vi "ADAM-4117_Log_ModbusRTU.NET.vi"() -> ()   [LabVIEW 2014]
uses:
  ModbusRTU/bin/Debug/Advantech.Adam.dll
  <vilib>/Platform/TimedLoop/XDataNode/timing_clust.ctl
  <vilib>/Platform/TimedLoop/XDataNode/nitl_modes.ctl
  <vilib>/Platform/TimedLoop/XDataNode/wakeup.ctl
  <vilib>/Platform/TimedLoop/XDataNode/XDataNode.xnode
  <vilib>/Platform/TimedLoop/XDataNode/XDNodeRunTimeDep.lvlib
panel:
  out "Waveform Chart":dbl(graph)
  out "ReadHoldingRegs":bool
  out "SetComPortTimeout":bool
  out "SetComPortState":bool
  out "OpenComPort":bool
  out "CloseComPort":bool
  in  "stop":bool
  in  "Address":i32=3
  in  "COM Port":i32=3
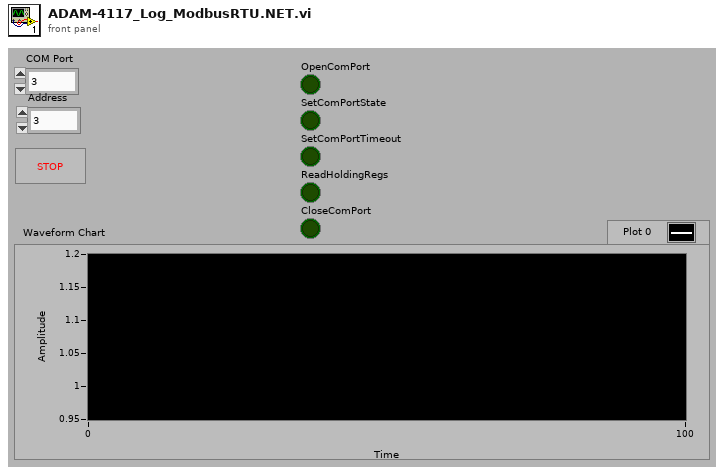
[diagram p1: front panel]
types:
  T1 = enum16{"open", "replace", "create", "open or create", "replace or create", "replace or create with confirmation"}
  T2 = typedef "XDNodeRunTimeDep.lvlib/timing_clust.ctl" = cluster{"Expected End [f-1]":u64, "Actual End [f-1]":u64, "Finished Late? [f-1]":bool, "Expected End [i-1]":u64, "Actual End [i-1]":u64, "Finished Late? [i-1]":bool, "Expected Start [i]":u64, "Actual Start [i]":u64, "Expected Start [f]":u64, "Actual Start [f]":u64, "Source Name":string, "Structure Name":string, "Period":i64, "Deadline":i64, "Offset":i64, "Start":i64, "Priority":i32, "Timeout":i32, "Mode":T3, "Wakeup Reason":T4, "Error":errorcluster, "Source Type":string, "Secondary Source Type":string, "Global End Time":u64, "Global Start Time":u64, "Frame Duration":u64, "Iteration Duration":u64, "Assigned CPU":i32, "I/O Scan Engine Mode":u32}
  T3 = typedef "XDNodeRunTimeDep.lvlib/nitl_modes.ctl" = enum32{"No Change", "Process missed periods, maintain original phase", "Discard missed periods, maintain original phase", "Process missed periods, ignore original phase", "Discard missed periods, ignore original phase"}
  T4 = typedef "XDNodeRunTimeDep.lvlib/wakeup.ctl" = enum32{"Normal", "Aborted", "Asynchronous wakeup", "Timing source error", "Timed loop error", "Timeout"}
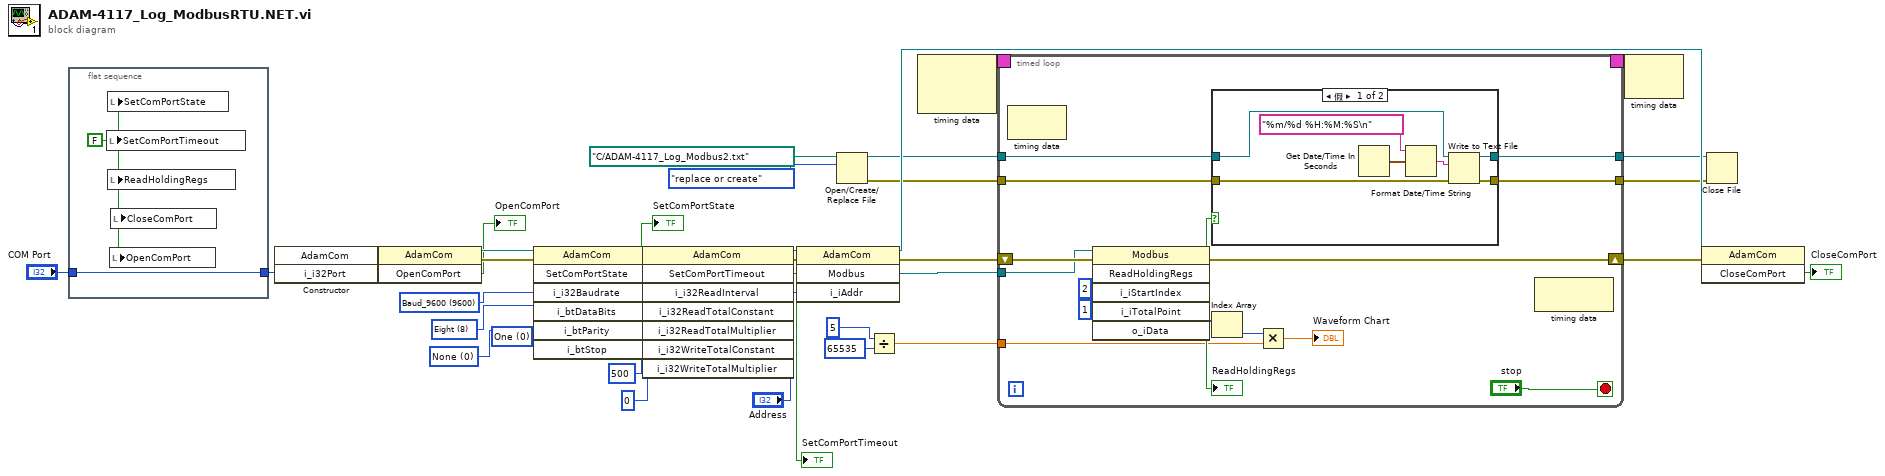
[diagram p0: block diagram]
diagram:
  w25 = 0 ("i_i32ReadTotalMultiplier")
  w26 = 500 ("i_i32ReadInterval")
  w29 = u8 0 items=["One", "OneAndHalf", "Two"] ("i_btStop")
  w30 = u8 0 items=["None", "Odd", "Even", "Mark", "Space"] ("i_btParity")
  w31 = u8 8 items=["Five"=5, "Six"=6, "Seven"=7, "Eight"=8] ("i_btDataBits")
  w32 = 9600 items=["Baud_110"=110, "Baud_300"=300, "Baud_600"=600, "Baud_1200"=1200, "Baud_2400"=2400, "Baud_4800"=4800, "Baud_9600"=9600, "Baud_14400"=14400, "Baud_19200"=19200, "Baud_38400"=38400, "Baud_56000"=56000, "Baud_57600"=57600, "Baud_115200"=115200, "Baud_128000"=128000, "Baud_256000"=256000] ("i_i32Baudrate")
  n1 = flat-sequence {
    tunnel: "COM Port" -> [w38]
    tunnel: [w38] -> w10
    frame #0 {
      w37 = FALSE
      n2 = local write "SetComPortTimeout"(w37) -> ()
      n3 = local write "SetComPortState"(w37) -> ()
      n4 = local write "ReadHoldingRegs"(w37) -> ()
      n5 = local write "OpenComPort"(w37) -> ()
      n6 = local write "CloseComPort"(w37) -> ()
    }
  }
  n7 = constructor class="AdamCom"("i_i32Port"=w10) -> (reference out=w36:refnum<k24>, error out=w35:errorcluster)  [unwired: 3 in, 2 out]
  n8 = invoke class="AdamCom" method="OpenComPort"(reference=w36, error in=w35) -> (reference out=w33:refnum<k24>, error out=w34:errorcluster, "OpenComPort"=→"OpenComPort":bool)  [unwired: 1 in]
  n9 = invoke class="AdamCom" method="SetComPortState"(reference=w33, error in=w34, "i_i32Baudrate"=w32, "i_btDataBits"=w31, "i_btParity"=w30, "i_btStop"=w29) -> (reference out=w27:refnum<k24>, error out=w28:errorcluster, "SetComPortState"=→"SetComPortState":bool)  [unwired: 1 in, 4 out]
  n10 = invoke class="AdamCom" method="SetComPortTimeout"(reference=w27, error in=w28, "i_i32ReadInterval"=w26, "i_i32ReadTotalConstant"=w26, "i_i32ReadTotalMultiplier"=w25, "i_i32WriteTotalConstant"=w26, "i_i32WriteTotalMultiplier"=w25) -> (reference out=w24:refnum<k24>, error out=w23:errorcluster, "SetComPortTimeout"=→"SetComPortTimeout":bool)  [unwired: 1 in, 5 out]
  n11 = invoke class="AdamCom" method="Modbus"(reference=w24, error in=w23, "i_iAddr"="Address") -> (reference out=w15:refnum<k24>, error out=w17:errorcluster, "Modbus"=w21:refnum<k24>)  [unwired: 1 in, 1 out]
  n12 = Open/Create/Replace File(file path (use dialog)=path "C:/ADAM-4117_Log_Modbus2.txt", operation (0:open)=T1."replace or create") -> (refnum out=w5:refnum<file>, error out=w7:errorcluster)  [unwired: 1 in, 4 out]
  n13 = Divide(x=5, y=65535) -> (x/y=w1:dbl)
  n14 = node-c288() -> (w20:T2)  [unwired: 2 out]
  n15 = timed-loop {
    timing: w20 -> [_]
    timing-out: [_] -> w19
    tunnel: w21 -> [w50]
    shift-right: [w51] -> w16
    shift-left: w17 -> [w52]
    tunnel: w7 -> [w46]
    tunnel: [w45] -> w6
    tunnel: w5 -> [w44]
    tunnel: [w43] -> w4
    tunnel: w1 -> [w40]
    stop <- "stop" stop-if-true
    n16 = node-c288() -> ()  [unwired: 2 out]
    n17 = invoke class="Modbus" method="ReadHoldingRegs"(reference=w50, error in=w52, "i_iStartIndex"=2, "i_iTotalPoint"=1) -> (error out=w51:errorcluster, "ReadHoldingRegs"=w42:bool, "o_iData"=w47:i32[])  [unwired: 2 in, 3 out]
    "ReadHoldingRegs" <- w42
    n18 = case shown="假" w42 {
      tunnel: w46 -> [w60 w62]
      tunnel: [w59 w62] -> w45
      tunnel: w44 -> [w58 w61]
      tunnel: [w57 w61] -> w43
      frame False {
        n19 = Get Date/Time In Seconds() -> (seconds since 1Jan1904=w54:timestamp)
        n20 = Format Date/Time String(time format string (%c)="%m/%d %H:%M:%S\n", seconds (now)=w54) -> (date/time string=w55:string)  [unwired: 1 out]
        n21 = Write to Text File(file (use dialog)=w58, text=w55, error in=w60) -> (refnum out=w57:refnum<file>, error out=w59:errorcluster)  [unwired: 2 out]
      }
      frame True {
      }
    }
    n22 = Index Array(array=w47) -> (element=w41:i32)  [unwired: 1 in]
    n23 = Multiply(x=w41, y=w40) -> (x*y=→"Waveform Chart":dbl)
    n24 = node-c288() -> ()  [unwired: 2 out]
  }
  n25 = node-c288(w19) -> ()  [unwired: 1 out]
  n26 = invoke class="AdamCom" method="CloseComPort"(reference=w15, error in=w16) -> ("CloseComPort"=→"CloseComPort":bool)  [unwired: 1 in, 2 out]
  n27 = Close File(refnum=w4, error in=w6) -> ()  [unwired: 2 out]
